vi "RSZVB Export Characterization Data to Touchstone Files.vi"(8 "error in (no error)":errorcluster {"code" format="%.0x"}, 10 "File Name":string, 11 "VISA session":refnum<visa-resource-name>) -> (0 "error out":errorcluster {"code" format="%.0x"}, 3 "dup VISA session":refnum<visa-resource-name>)   [LabVIEW 2011]
doc: "This VI exports the calibration unit's characterization data as Touchstone files into the given directory.\n\nRemote-control command(s):\n:MMEMory:AKAL:FACTory:CONVersion <file_name>"
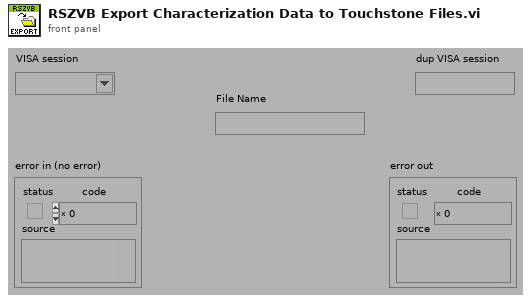
[diagram p1: front panel]
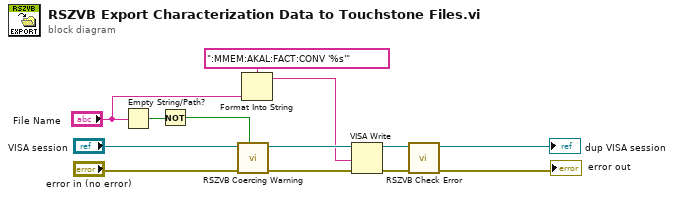
[diagram p0: block diagram]
diagram:
  n1 = Empty String/Path?(string/path="File Name") -> (empty?=w3:bool)
  n2 = Not(x=w3) -> (.not. x?=w2:bool)
  n3 = call "RSZVB Coercing Warning.vi"("In Range?"=w2, "error in (no error)"="error in (no error)", "VISA session"="VISA session") -> ("error out"=w12:errorcluster, "dup VISA session"=w13:refnum<visa-resource-name>)  [unwired: 7 in]
  n4 = Format Into String(format string=":MMEM:AKAL:FACT:CONV '%s'", "File Name") -> (resulting string=w6:string)  [unwired: 2 in, 1 out]
  n5 = VISA Write(VISA resource name=w13, write buffer=w6, error in (no error)=w12) -> (VISA resource name out=w10:refnum<visa-resource-name>, error out=w11:errorcluster)  [unwired: 1 out]
  n6 = call "RSZVB Check Error.vi"("error in (no error)"=w11, "VISA session"=w10) -> ("error out"=→"error out":errorcluster, "dup VISA session"=→"dup VISA session":refnum<visa-resource-name>)  [unwired: 8 in]
